vi "save VTK File.vi"(8 "error in (no error)":errorcluster, 11 "path":string) -> (0 "error out":errorcluster)   [LabVIEW 2019, in "libConvectionDiffusionWrapper.lvlib"]
doc: "void saveVTKFile(const char* path);"
uses:
  libConvectionDiffusionWrapper.lvlib
  libConvectionDiffusionWrapper.so
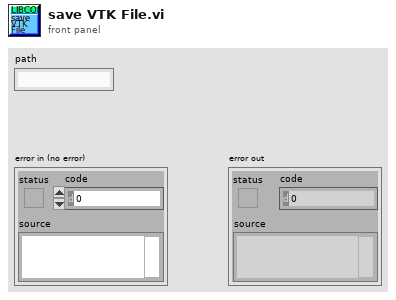
[diagram p1: front panel]
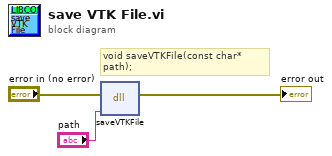
[diagram p0: block diagram]
diagram:
  # "void saveVTKFile(const char* path);"
  n1 = dll-call lib="home/paul/Schreibtisch/Convection_diffusion/LabView/lib/libConvectionDiffusionWrapper.*" fn="saveVTKFile"(error in="error in (no error)", "path"="path") -> (error out=→"error out":errorcluster)  [unwired: 4 in, 1 out]
